vi "Firewall State'.vi"(8 "error in (no error)":errorcluster) -> (0 "error out":errorcluster, 3 "Firewall On":bool)   [LabVIEW 2020]
uses:
  <vilib>/registry/registry.llb/Registry SAM.ctl
  <vilib>/registry/registry.llb/Registry RtKey.ctl
  <vilib>/registry/registry.llb/Read Registry Value Simple U32.vi
panel:
  out "DWORD data":u32
  out "values":string[](array[string])
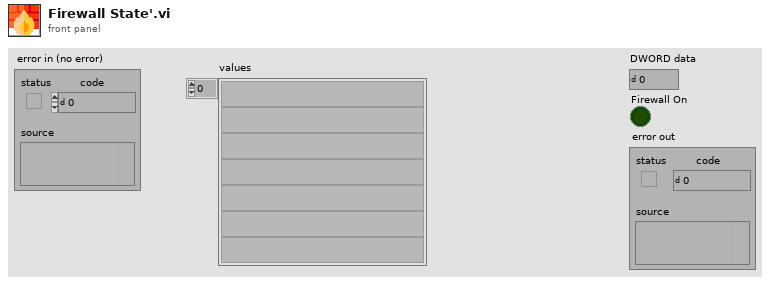
[diagram p1: front panel]
types:
  T1 = typedef "Registry RtKey.ctl" = enum32{"HKEY_CLASSES_ROOT", "HKEY_CURRENT_USER", "HKEY_LOCAL_MACHINE", "HKEY_USERS", "HKEY_PERFORMANCE_DATA", "HKEY_CURRENT_CONFIG", "HKEY_DYN_DATA"}
  T2 = typedef "Registry SAM.ctl" = enum32{"KEY_QUERY_VALUE", "KEY_SET_VALUE", "KEY_CREATE_SUB_KEY", "KEY_ENUMERATE_SUB_KEYS", "KEY_NOTIFY", "KEY_CREATE_LINK", "KEY_READ", "KEY_WRITE", "KEY_ALL_ACCESS", "KEY_READ | KEY_WRITE"}
  T3 = typedef "Registry refnum.ctl" = refnum<k1>
  T4 = cluster{"numValues":i32, "maxValueNameLen":i32, "maxValueDataLen":i32}
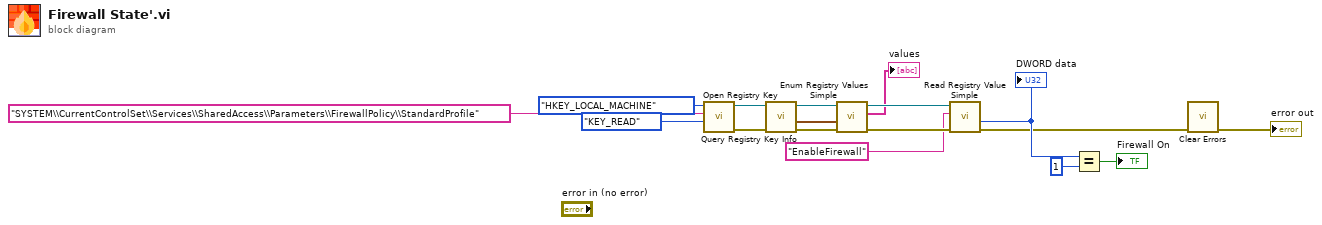
[diagram p0: block diagram]
diagram:
  n1 = call <vilib>:"Open Registry Key.vi"("security access mask (KEY_READ | KEY_WRITE)"=Registry_SAM."KEY_READ", "subkey"="SYSTEM\\CurrentControlSet\\Services\\SharedAccess\\Parameters\\FirewallPolicy\\StandardProfile", "root key (HKEY_LOCAL_MACHINE)"=Registry_RtKey."HKEY_LOCAL_MACHINE") -> ("error out"=w11:errorcluster, "refnum out"=w12:T3)  [unwired: 7 in]
  n2 = call <vilib>:"Query Registry Key Info.vi"("error in (no error)"=w11, "refnum"=w12) -> ("error out"=w15:errorcluster, "value info"=w14:T4, "refnum out"=w13:T3)  [unwired: 5 in, 2 out]
  n3 = call <vilib>:"Enum Registry Values Simple.vi"("error in (no error)"=w15, "value info"=w14, "refnum"=w13) -> ("error out"=w9:errorcluster, "values"=→"values":string[], "refnum out"=w10:T3)  [unwired: 3 in, 3 out]
  n4 = call-poly <vilib>:"Read Registry Value Simple.vi"("error in (no error)"=w9, "value"="EnableFirewall" ("value name"), "refnum"=w10) -> ("error out"=w2:errorcluster, "DWORD data"=w5:u32)  [unwired: 3 in, 2 out]
  "DWORD data" <- w5
  n5 = Equal?(x=w5, y=u32 1) -> (x = y?=→"Firewall On":bool)
  n6 = call <vilib>:"Clear Errors.vi"("error in (no error)"=w2) -> ("error out"=→"error out":errorcluster)  [unwired: 5 in, 1 out]
